vi "remove_edge.vi"(10 "edge":refnum<class "Edge.lvclass">, 11 "graph":refnum<class "Graph.lvclass">) -> (2 "key not found?":bool, 3 "graph out":refnum<class "Graph.lvclass">)   [LabVIEW 2020, in "graph.lvlib" / "Graph.lvclass"]
uses:
  Graph.lvclass
  Graph.lvclass/Graph.ctl
  Edge/Edge.lvclass
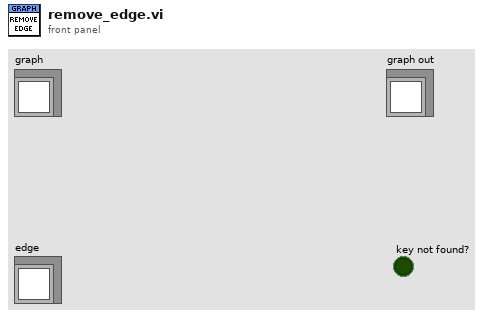
[diagram p1: front panel]
types:
  T1 = typedef "graph.lvlib/Graph.lvclass/edge-definition-cluster.ctl" = cluster{"source-id":refnum<class "ID.lvclass">, "sink-id":refnum<class "ID.lvclass">}
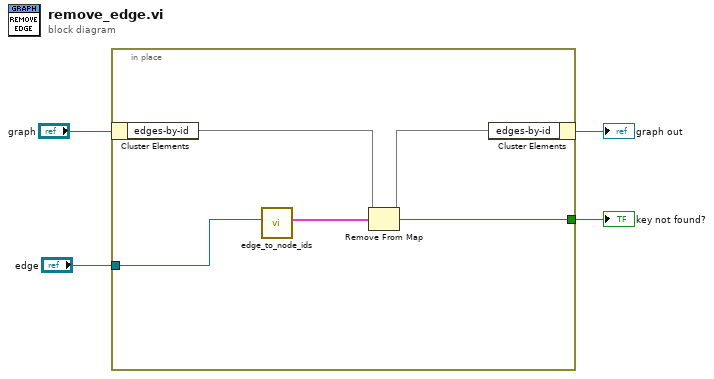
[diagram p0: block diagram]
diagram:
  n1 = in-place {
    in-place-border: [w5] -> w1
    in-place-border: "edge" -> [w9]
    n2 = in-place-cluster #1("graph") -> ("edges-by-id"=w8:map{T1, refnum<class "Edge.lvclass">})
    n3 = call "edge_to_node_ids.vi"("edge"=w9) -> ("node-ids-cluster"=w6:T1)  [unwired: 10 in]
    n4 = Remove From Map(10:w6, 11:w8) -> (2:w5:bool, 3:w7:map{T1, refnum<class "Edge.lvclass">})  [unwired: 1 out]
    n5 = in-place-cluster #1("edges-by-id"=w7) -> (→"graph out":refnum<class "Graph.lvclass">)
  }
  "key not found?" <- w1
